vi "setAttributeTreeValue_action.vi"(0 "HGF_ImaqDx":refnum<class "HGF_ImaqDx.lvclass">, 1 "Tree Control In":refnum<vi>, 3 "Tab Control Ref In":T1, 5 "error in (no error)":errorcluster) -> (14 "dup HGF_ImaqDx":refnum<class "HGF_ImaqDx.lvclass">, 15 "Tree Control Out":refnum<vi>, 19 "error out":errorcluster)   [LabVIEW 2014, in "HGF_IMAQ.lvlib" / "HGF_ImaqDx.lvclass"]
doc: "This is the override VI to set cameras selected attribute value."
uses:
  HGF_ImaqDx.lvclass
  VisionTools/HGF_VisionTools/HGF_VisionTools.lvlib
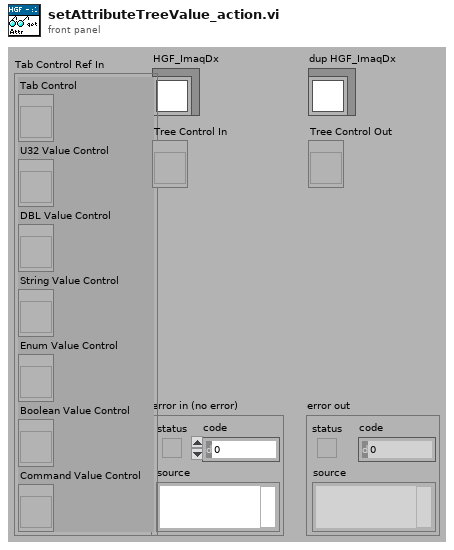
[diagram p1: front panel]
types:
  T1 = cluster{"Tab Control":refnum<vi>, "U32 Value Control":refnum<vi>, "DBL Value Control":refnum<vi>, "String Value Control":refnum<vi>, "Enum Value Control":refnum<vi>, "Boolean Value Control":refnum<vi>, "Command Value Control":refnum<vi>}
  T2 = typedef "IMAQdx.ctl" = refnum<k21>
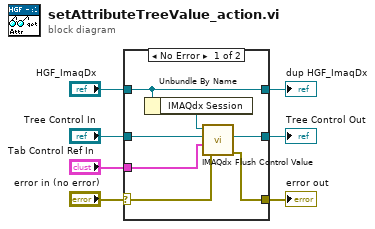
[diagram p0: block diagram]
diagram:
  n1 = case shown="No Error" "error in (no error)" {
    selector: "error in (no error)" -> [w9 w16]
    tunnel: [w14 w17] -> w6
    tunnel: "HGF_ImaqDx" -> [w14 w17]
    tunnel: [w8 w16] -> w4
    tunnel: [w12 w15] -> w3
    tunnel: "Tree Control In" -> [w13 w15]
    tunnel: "Tab Control Ref In" -> [w10 _]
    frame No Error {
      n2 = Unbundle By Name(w14) -> ("IMAQdx Session"=w11:T2)
      n3 = call "IMAQdx Flush Control Value.vi"("error in (no error)"=w9, "Tab Control Ref In"=w10, "Tree Control In"=w13, "Session In"=w11) -> ("error out"=w8:errorcluster, "Tree Control Out"=w12:refnum<vi>)  [unwired: 2 out]
    }
    frame Error {
    }
  }
  "error out" <- w4
  "dup HGF_ImaqDx" <- w6
  "Tree Control Out" <- w3
